vi "5FT.vi"(1 "Camera Instance":T1(plugin-control), 7 "error in":errorcluster) -> (20 "Matches (Geometric Matching 1)":T2[](array[typedef]) {"Correlation Score" format="%.2f"; "Target Template Curve Score" format="%.2f"; "Template Target Curve Score" format="%.2f"; "Bounding Box"."y" format="%.2f"; "Bounding Box"."x" format="%.2f"; "Position"."y" format="%.2f"; "Position"."x" format="%.2f"; "Score" format="%.2f"; "Scale" format="%.2f"; "Angle" format="%.2f"; "Occlusion %" format="%.2f"}, 21 "Calibrated Matches (Geometric Matching 1)":T2[](array[typedef]) {"Correlation Score" format="%.2f"; "Target Template Curve Score" format="%.2f"; "Template Target Curve Score" format="%.2f"; "Bounding Box"."y" format="%.2f"; "Bounding Box"."x" format="%.2f"; "Position"."y" format="%.2f"; "Position"."x" format="%.2f"; "Score" format="%.2f"; "Scale" format="%.2f"; "Angle" format="%.2f"; "Occlusion %" format="%.2f"}, 22 "Number of Matches (Geometric Matching 1)":i32, 24 "Instance Out":T1(plugin-control), 27 "error out":errorcluster)   [LabVIEW 2016]
uses:
  <vilib>/vision/Pattern Matching.llb/IMAQ GM Match Report.ctl
  <vilib>/vision/Image Controls.llb/Vision Info Type2.ctl
  <vilib>/vision/Pattern Matching.llb/IMAQ Curve Parameters.ctl
  <vilib>/vision/Pattern Matching.llb/IMAQ Match Range Setting.ctl
  <vilib>/vision/NI_Vision_Development_Module.lvlib
panel:
  out "Image Out":T1(plugin-control)
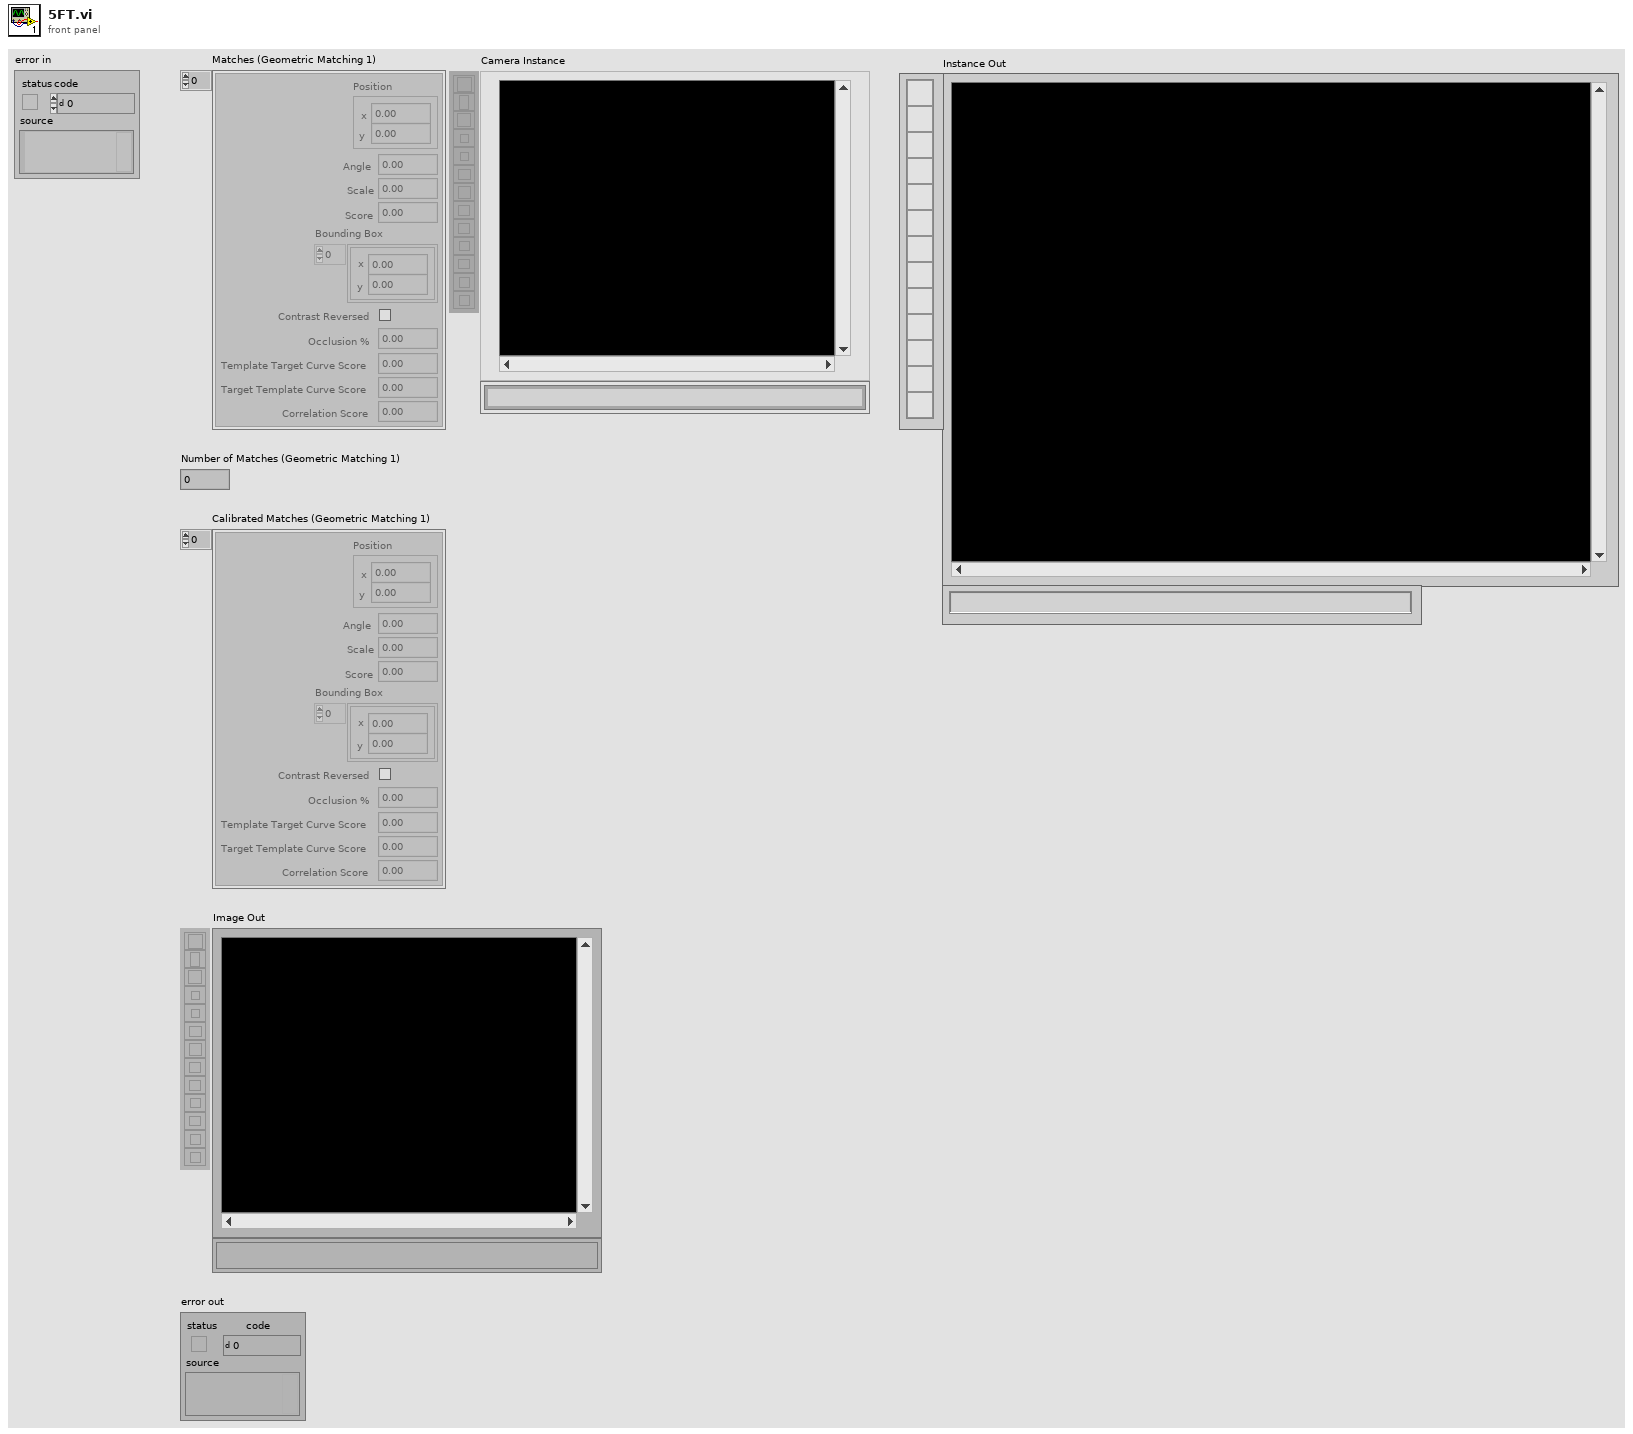
[diagram p1: front panel]
types:
  T1 = typedef "IMAQ Image.ctl" = refnum<image>
  T2 = typedef "IMAQ GM Match Report.ctl" = cluster{"Position":cluster{"x":sgl, "y":sgl}, "Angle":sgl, "Scale":sgl, "Score":sgl, "Bounding Box":cluster{"x":sgl, "y":sgl}[], "Contrast Reversed":bool, "Occlusion %":sgl, "Template Target Curve Score":sgl, "Target Template Curve Score":sgl, "Correlation Score":sgl}
  T3 = typedef "IMAQ Curve Parameters.ctl" = cluster{"Extraction Mode":u32, "Edge Threshold":i32, "Edge Filter Size":u32, "Min Length":i32, "Row Search Step Size":i32, "Col Search Step Size":i32, "Max Endpoint Gap":i32, "Closed":bool, "Subpixel":bool}
  T4 = typedef "IMAQ Match Range Setting.ctl" = cluster{"Match Constraints":u32, "Min":dbl, "Max":dbl}
  T5 = cluster{"Curve Parameters":T3, "Match Mode":cluster{"Rotation":bool, "Scale":bool, "Occlusion":bool, "Reserved":bool, "Reserved":bool, "Reserved":bool}, "Range Settings":T4[], "Number of Matches":i32, "Minimum Match Score":sgl, "SubPixel Accuracy":bool, "Adv. Geometric Match Options 2":cluster{"Setup Data Item":u16, "Item Value":dbl}[]}
  T6 = cluster{"Global Rectangle":i32[], "Contours":cluster{"ID":enum32{"External", "Internal"}, "Type":u32, "Coordinates":i32[]}[]}
  T7 = typedef "Vision Info Type2.ctl" = u32
  T8 = cluster{"Origin Pixel":cluster{"X":sgl, "Y":sgl}, "Angle Relative to Horizontal (deg)":sgl, "Axis Reference":u32}
  T9 = enum32{"AutoM", "Close", "Dilate", "Erode", "Gradient", "Gradient out", "Gradient in", "Hit miss", "Open", "PClose", "POpen", "Thick", "Thin"}
  T10 = cluster{"Brightness":sgl, "Contrast":sgl, "Gamma":sgl}
  T11 = cluster{"histogram":u32[], "Minimal Value":sgl, "Maximal Value":sgl, "Starting Value":sgl, "Interval Width":sgl, "Mean Value":sgl, "Standard  Variation":sgl, "Area (pixels)":i32}
  T12 = typedef "Image Type" = u32
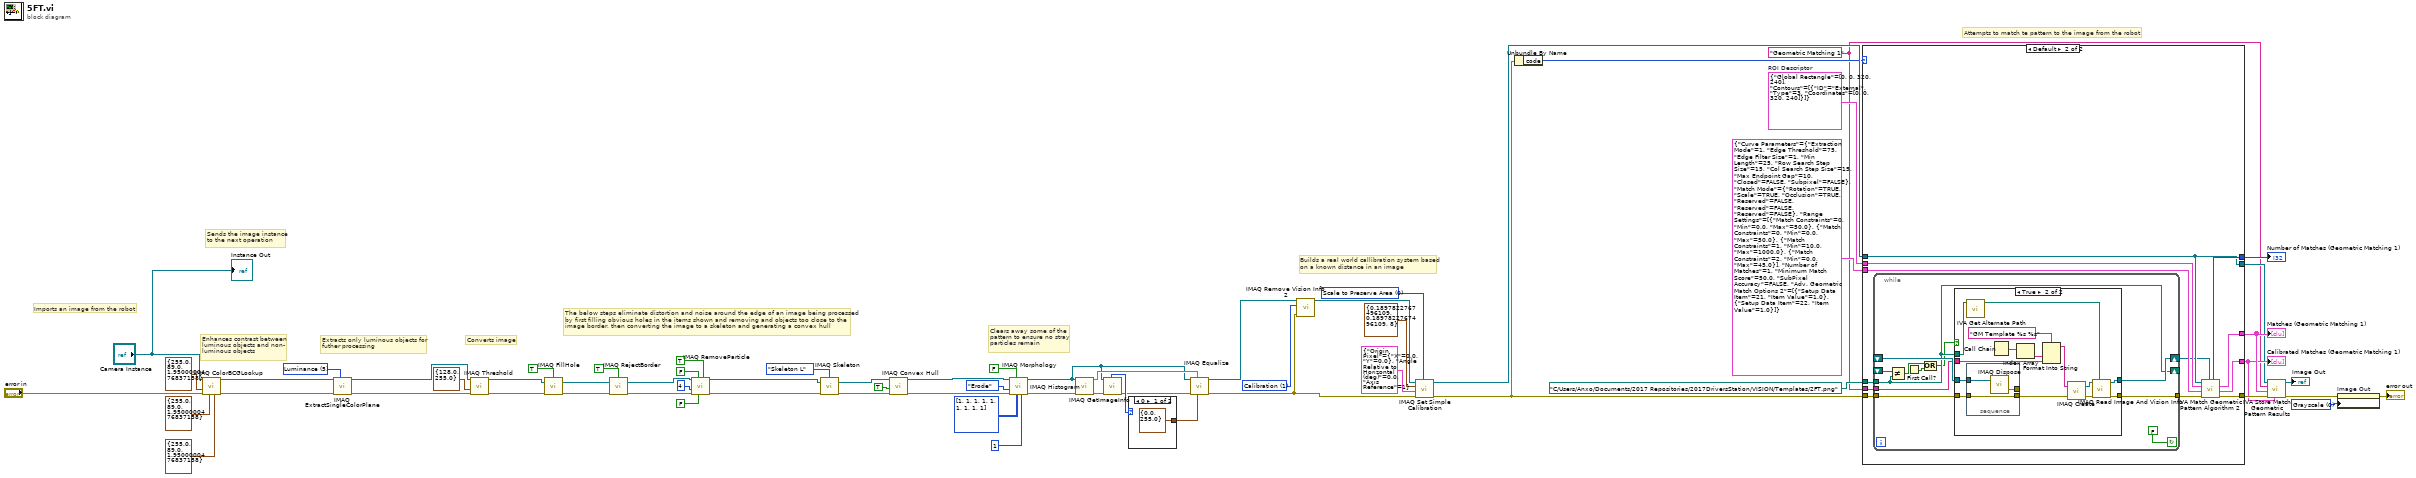
[diagram p0: block diagram]
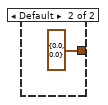
[diagram p4: hidden frame]
diagram:
  w3 = u32 0 items=["Grayscale", "Binary", "Gradient", "Rainbow", "Temperature", "User Defined", "Binary 16 Bit", "Gradient 16 Bit", "Rainbow 16 Bit", "Temperature 16 Bit", "User Defined 16 Bit"] ("Palette Type")
  w7 = "Geometric Matching 1" ("Step Name")
  w17 = T6 {"Global Rectangle"=[0, 0, 320, 240], "Contours"=[{"ID"=enum."External", "Type"=3, "Coordinates"=[0, 0, 320, 240]}]}  # ROI Descriptor
  w20 = T7 1 items=["Any", "Calibration", "Overlay", "Grayscale Template", "Color Template", "Geometric Template", "Custom Data", "Golden Template", "Geometric Template 2", "Contour Data", "Camera Model"] ("Vision Info")
  w25 = u32 0 items=["Scale to Preserve Area", "Scale to Fit"] ("Corrected Image Scaling")
  w62 = 5 items=["Red", "Green", "Blue", "Hue", "Saturation", "Luminance", "Value", "Intensity"] ("Color Plane")
  # "Sends the image instance\nto the next operation"
  # "Attempts to match te pattern to the image from the robot"
  # "Builds a real world callibration system based\non a known distance in an image"
  # "Clears away some of the \npattern to ensure no stray\nparticles remain"
  # "The below steps eliminate distortion and noise around the edge of an image being processed\nby first filling obvious holes in the items shown and removing and objects too close to the\nimage border, then converting the image to a skeleton and generating a convex hull"
  # "Converts image"
  # "Extracts only luminous objects for\nfuther processing"
  # "Enhances contrast between\nluminous objects and non-\nluminous objects"
  # "Imports an image from the robot"
  n1 = call "IMAQ ColorBCGLookup"("Blue BCG Values"=T10 {"Brightness"=255.0, "Contrast"=89.0, "Gamma"=1.95}, "Green BCG Values"=T10 {"Brightness"=255.0, "Contrast"=89.0, "Gamma"=1.95}, "error in (no error)"="error in", "Red BCG Values"=T10 {"Brightness"=255.0, "Contrast"=89.0, "Gamma"=1.95}, "Image Src"="Camera Instance") -> ("error out"=w60:errorcluster, "Image Dst Out"=w61:T1)  [unwired: 2 in, 3 out]
  n2 = call "IMAQ ExtractSingleColorPlane"("Color Plane"=w62, "error in (no error)"=w60, "Image Src"=w61) -> ("error out"=w57:errorcluster, "Image Dst Out"=w58:T1)  [unwired: 1 in, 6 out]
  n3 = call "IMAQ Threshold"("error in (no error)"=w57, "Range"=cluster{"Lower value":sgl, "Upper value":sgl} {"Lower value"=128.0, "Upper value"=255.0}, "Image Src"=w58) -> ("error out"=w54:errorcluster, "Image Dst Out"=w55:T1)  [unwired: 3 in, 4 out]
  n4 = call "IMAQ FillHole"("error in (no error)"=w54, "Image Src"=w55, "Connectivity 4/8 (8)"=TRUE) -> ("error out"=w51:errorcluster, "Image Dst Out"=w52:T1)  [unwired: 1 in, 2 out]
  n5 = call "IMAQ RejectBorder"("error in (no error)"=w51, "Image Src"=w52, "Connectivity 4/8 (8)"=TRUE) -> ("error out"=w45:errorcluster, "Image Dst Out"=w46:T1)  [unwired: 1 in, 2 out]
  n6 = call "IMAQ RemoveParticle"("Connectivity 4/8 (8)"=TRUE, "Low Pass/High Pass (Low)"=FALSE, "Square/Hexa (Square)"=FALSE, "error in (no error)"=w45, "Number of Erosion"=4, "Image Src"=w46) -> ("error out"=w42:errorcluster, "Image Dst Out"=w43:T1)  [unwired: 1 in, 3 out]
  n7 = call "IMAQ Skeleton"("error in (no error)"=w42, "Image Src"=w43, "Mode"=enum32{"Skeleton L", "Skeleton M", "Skiz"}."Skeleton L") -> ("error out"=w40:errorcluster, "Image Dst Out"=w41:T1)  [unwired: 1 in, 2 out]
  n8 = call "IMAQ Convex Hull"("error in (no error)"=w40, "Connectivity 4/8 (8)"=TRUE, "Image Src"=w41) -> ("error out"=w33:errorcluster, "Image Dst Out"=w34:T1)  [unwired: 1 in, 6 out]
  n9 = call "IMAQ Morphology"("Number of iterations (1)"=1, "Structuring Element"=i32[][] [[1, 1, 1], [1, 1, 1], [1, 1, 1]], "Square/Hexa (Square)"=FALSE, "error in (no error)"=w33, "Operation"=T9."Erode", "Image Src"=w34) -> ("error out"=w31:errorcluster, "Image Dst Out"=w29:T1)  [unwired: 1 in, 3 out]
  n10 = call "IMAQ Histogram"("error in (no error)"=w31, "Image"=w29) -> ("error out"=w28:errorcluster, "Histogram Report"=w32:T11)  [unwired: 3 in, 5 out]
  n11 = call "IMAQ GetImageInfo"("error in (no error)"=w28, "Image"=w29) -> ("error out"=w27:errorcluster, "Image Type"=w30:T12)  [unwired: 8 out]
  n12 = case shown="0" w30 {
    tunnel: [cluster{"Minimum":sgl, "Maximum":sgl} {"Minimum"=0.0, "Maximum"=255.0} ("Range") cluster{"Minimum":sgl, "Maximum":sgl} {"Minimum"=0.0, "Maximum"=0.0} ("Range")] -> w26
    frame 0 {
    }
    frame Default {
    }
  }
  n13 = call "IMAQ Equalize"("Range"=w26, "Histogram Report"=w32, "error in (no error)"=w27, "Image Src"=w29) -> ("error out"=w19:errorcluster, "Image Dst Out"=w22:T1)  [unwired: 2 in, 4 out]
  n14 = call "IMAQ Remove Vision Info 2"("error in (no error)"=w19, "Vision Info"=w20, "Image"=w22) -> ("Image Out"=w21:T1)  [unwired: 8 out]
  n15 = call "IMAQ Set Simple Calibration"("Corrected Image Scaling"=w25, "error in (no error)"=w19, "Calibration Axis Info"=T8 {"Origin Pixel"={"X"=0.0, "Y"=0.0}, "Angle Relative to Horizontal (deg)"=0.0, "Axis Reference"=1}, "Grid Descriptor"=cluster{"X Step":sgl, "Y Step":sgl, "Unit":u32} {"X Step"=0.18978228, "Y Step"=0.18978228, "Unit"=8}, "Image"=w21) -> ("error out"=w11:errorcluster, "Calibrated Image"=w16:T1)  [unwired: 1 in, 4 out]
  n16 = Unbundle By Name(w11) -> ("code"=w10:i32)
  n17 = case shown="Default" w10 {
    tunnel: path "C:/Users/Anxo/Documents/2017 Repositories/2017DriversStation/VISION/Templates/2FT.png" ("Template File Path") -> [_ w73]
    tunnel: w11 -> [_ w72]
    tunnel: T5 {"Curve Parameters"={"Extraction Mode"=1, "Edge Threshold"=75, "Edge Filter Size"=1, "Min Length"=25, "Row Search Step Size"=15, "Col Search Step Size"=15, "Max Endpoint Gap"=10, "Closed"=FALSE, "Subpixel"=FALSE}, "Match Mode"={"Rotation"=TRUE, "Scale"=TRUE, "Occlusion"=TRUE, "Reserved"=FALSE, "Reserved"=FALSE, "Reserved"=FALSE}, "Range Settings"=[{"Match Constraints"=0, "Min"=0.0, "Max"=50.0}, {"Match Constraints"=0, "Min"=0.0, "Max"=50.0}, {"Match Constraints"=1, "Min"=10.0, "Max"=1000.0}, {"Match Constraints"=2, "Min"=0.0, "Max"=45.0}], "Number of Matches"=1, "Minimum Match Score"=50.0, "SubPixel Accuracy"=FALSE, "Adv. Geometric Match Options 2"=[{"Setup Data Item"=21, "Item Value"=1.0}, {"Setup Data Item"=22, "Item Value"=1.0}]} ("Settings") -> [_ w80]
    tunnel: w17 -> [_ w79]
    tunnel: w16 -> [w68 w74]
    tunnel: [_ w78] -> w15
    tunnel: [_ w77] -> w14
    tunnel: [_ w76] -> w13
    tunnel: [_ w75] -> w12
    tunnel: [w68 w74] -> w9
    tunnel: w7 -> [_ w69]
    frame -1074396199, -1074396198 {
      # "Discard Coordinate System Error"
    }
    frame Default {
      n18 = while {
        shift-right: [w91] -> w70
        shift-left: _ -> [w90]
        tunnel: [w88] -> w71
        tunnel: w72 -> [w87]
        tunnel: w73 -> [w84]
        tunnel: w69 -> [w86]
        shift-right: [w84] -> _
        shift-left: _ -> [w85]
        stop <- FALSE continue-if-true
        n19 = Not Equal?(x=w85, y=w84) -> (x != y?=w82:bool)
        n20 = First Call?() -> (First Call?: T/F=w83:bool)
        n21 = Or(x=w82, y=w83) -> (x .or. y?=w81:bool)
        n22 = case shown="True" w81 {
          tunnel: [w93 w105] -> w91
          tunnel: w90 -> [w93 w97]
          tunnel: [w92 w102] -> w88
          tunnel: w87 -> [w92 w98]
          tunnel: w86 -> [_ w99]
          tunnel: w84 -> [_ w95]
          frame False {
          }
          frame True {
            n23 = call <vilib>:"IVA Get Alternate Path.vi"("Path In"=w95) -> ("Path Out"=w94:path)  [unwired: 10 out]
            n24 = stacked-sequence {
              tunnel: w98 -> [w110]
              tunnel: w97 -> [w109]
              tunnel: [w110] -> w96
              tunnel: [w108] -> _
              frame #0 {
                n25 = call "IMAQ Dispose"("Image"=w109) -> ("error out"=w108:errorcluster)  [unwired: 2 in, 3 out]
              }
            }
            n26 = Call Chain() -> (call chain=w101:string[])
            n27 = Index Array(array=w101) -> (element=w100:string)  [unwired: 1 in]
            n28 = Format Into String(format string="GM Template %s %s" ("Image Name"), w100, w99) -> (resulting string=w107:string)  [unwired: 2 in, 1 out]
            n29 = call "IMAQ Create"("Image Name"=w107, "error in (no error)"=w96) -> ("New Image"=w104:T1, "error out"=w103:errorcluster)  [unwired: 2 in, 1 out]
            n30 = call "IMAQ Read Image And Vision Info"("File Path"=w94, "error in (no error)"=w103, "Image"=w104) -> ("error out"=w102:errorcluster, "Image Out"=w105:T1)  [unwired: 1 in, 6 out]
          }
        }
      }
      n31 = call <vilib>:"IVA Match Geometric Pattern Algorithm 2.vi"("Template"=w70, "error in (no error)"=w71, "Settings"=w80, "ROI Descriptor"=w79, "Image"=w74) -> ("error out"=w78:errorcluster, "Calibrated Matches"=w76:T2[], "Matches"=w77:T2[], "Number of Matches"=w75:i32)  [unwired: 1 in, 2 out]
    }
  }
  "Matches (Geometric Matching 1)" <- w14
  "Number of Matches (Geometric Matching 1)" <- w12
  "Calibrated Matches (Geometric Matching 1)" <- w13
  n32 = call <vilib>:"IVA Store Match Geometric Pattern Results.vi"("Calibrated Matches"=w13, "error in (no error)"=w15, "Matches"=w14, "Step Name"=w7, "Image in"=w9) -> ("error out"=w6:errorcluster, "Image dup"=→"Image Out":T1)  [unwired: 5 out]
  n33 = property on="Image Out" class="ImageControl"(error in=w6, "Palette:Palette Type"=w3) -> (error out=→"error out":errorcluster)  [unwired: 1 in, 1 out]
  "Instance Out" <- "Camera Instance"
